vi "Generate Random Gene.vi"(8 "error in":errorcluster, 11 "Object Gene in":refnum<class "Object Gene.lvclass">) -> (0 "error out":errorcluster, 3 "Object Gene out":refnum<class "Object Gene.lvclass">)   [LabVIEW 2016, in "Object Gene.lvclass"]
uses:
  Object Gene.lvclass
  IGene.lvclass
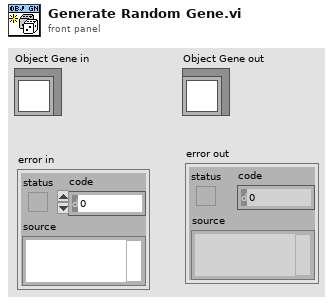
[diagram p1: front panel]
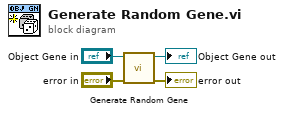
[diagram p0: block diagram]
diagram:
  n1 = call-parent "Generate Random Gene.vi"("error in"="error in", "IGene in"="Object Gene in") -> ("error out"=→"error out":errorcluster, "IGene out"=→"Object Gene out":refnum<class "Object Gene.lvclass">)  [unwired: 8 in]
